vi "Instance.vi"() -> (3 "App":refnum<class "App.lvclass">)   [LabVIEW 2020, in "App.lvclass"]
uses:
  App.lvclass
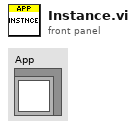
[diagram p1: front panel]
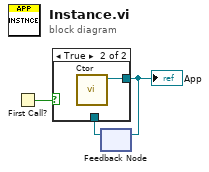
[diagram p0: block diagram]
diagram:
  n1 = First Call?() -> (First Call?: T/F=w3:bool)
  n2 = feedback #1() -> (w1:refnum<class "App.lvclass">)  [unwired: 1 in]
  n3 = case shown="True" w3 {
    tunnel: [w4 w5] -> w2
    tunnel: w1 -> [w4 _]
    frame False {
    }
    frame True {
      n4 = call "Ctor.vi"() -> ("App out"=w5:refnum<class "App.lvclass">)  [unwired: 10 in, 1 out]
    }
  }
  "App" <- w2
  n5 = feedback-in #1(w2) -> ()
